vi "ExistConfigFile.vi"(11 "file name":string) -> (2 "dup path":path caption="경로 복제", 3 "file or folder exists?":bool caption="파일 또는 폴더가 존재합니까?")   [LabVIEW 2018]
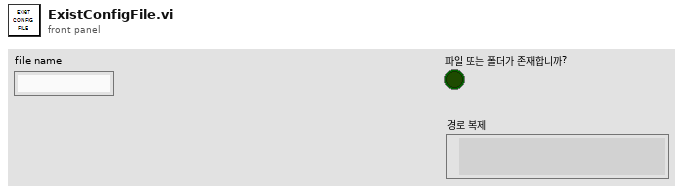
[diagram p1: front panel]
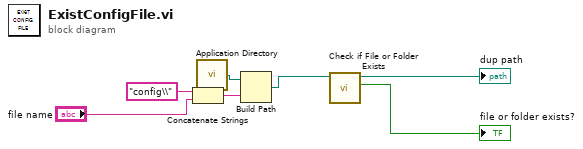
[diagram p0: block diagram]
diagram:
  n1 = Concatenate Strings("config\\" ("문자열"), "file name") -> (w5:string)
  n2 = call <vilib>:"Application Directory.vi"() -> ("Application Directory"=w4:path)
  n3 = Build Path(base path=w4, name or relative path=w5) -> (appended path=w3:path)
  n4 = call <vilib>:"Check if File or Folder Exists.vi"("path"=w3) -> ("file or folder exists?"=→"file or folder exists?":bool, "dup path"=→"dup path":path)  [unwired: 8 in, 1 out]
